vi "Gyro.vi"(1 "Reset Gyro":bool) -> (0 "Yaw Angle":dbl)   [LabVIEW 2018]
uses:
  <vilib>/Rock Robotics/WPI/ThirdParty/Phoenix-LabVIEW/Pigeon IMU/CTRE_PigeonIMU_TareType.ctl
  <vilib>/Rock Robotics/WPI/ThirdParty/Phoenix-LabVIEW/Pigeon IMU/CTRE_PigeonIMU_GetYPR.vi
  <vilib>/Rock Robotics/Network Tables/NT Write Number.vi
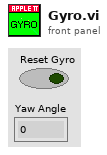
[diagram p1: front panel]
types:
  T1 = typedef "CTRE_PigeonIMU_DeviceRef.ctl" = cluster{"DeviceStatus":errorcluster, "Device Number":u8, "Type":T2, "Device ID":u32, "Handle":u64, "UsageFrame":u32, "Library Path":path}
  T2 = typedef "CTRE_PigeonIMU_ConnectionType.ctl" = u32
  T3 = typedef "CTRE_PigeonIMU_TareType.ctl" = u8
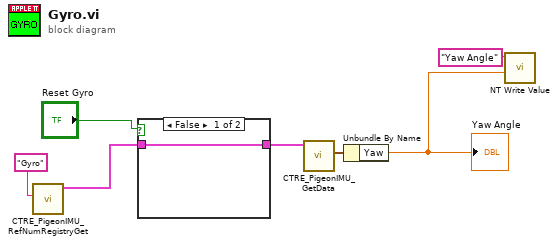
[diagram p0: block diagram]
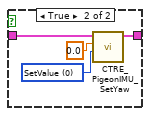
[diagram p2: hidden frame]
diagram:
  n1 = call <vilib>:"CTRE_PigeonIMU_RefNumRegistryGet.vi"("refnum name"="Gyro") -> ("PigeonIMUDevRef"=w2:T1)  [unwired: 9 in, 1 out]
  n2 = case shown="False" "Reset Gyro" {
    tunnel: [w8 w12] -> w6
    tunnel: w2 -> [w8 w9]
    frame False {
    }
    frame True {
      w11 = T3 0 items=["SetValue"=0, "AddOffset"=1, "MatchCompass"=2, "SetOffset"=255] ("TareType (SetValue)")
      n3 = call <vilib>:"CTRE_PigeonIMU_SetYaw.vi"("TareType (SetValue)"=w11, "Value"=0.0, "PigeonIMUDevRef"=w9) -> ("PigeonIMUDevRef"=w12:T1)  [unwired: 7 in, 1 out]
    }
  }
  n4 = call-poly <vilib>:"CTRE_PigeonIMU_GetData.vi"("PigeonIMUDevRef"=w6) -> ("Yaw Pitch Roll"=w7:cluster{"Yaw":dbl, "Pitch":dbl, "Roll":dbl})  [unwired: 8 in, 2 out]
  n5 = Unbundle By Name(w7) -> ("Yaw"=w1:dbl)
  "Yaw Angle" <- w1
  n6 = call-poly <vilib>:"NT Write Value.vi"("Numeric"=w1, "Name"="Yaw Angle") -> ()  [unwired: 9 in, 1 out]
